vi "Running Wrapper.vi"(8 "error in (no error)":errorcluster, 11 "CIFCorePlugin in":refnum<class "CIFCorePlugin.lvclass">) -> (0 "error out":errorcluster, 2 "Destroy":bool, 3 "CIFCorePlugin out":refnum<class "CIFCorePlugin.lvclass">)   [LabVIEW 2021, in "CIFCorePlugin.lvclass"]
doc: "Wrapper around the Core Running VI. This wrapper will handle selection of timed loop with priorities or execution without a timed loop. \n\nIf the VI is compiled to run on LinuxRT it will check if timed loop is supported (RT compiled PPLs can run on desktop but timed loop is not supported and conditional compile will not check after PPL is compiled). If the timed loop is supported it will check if the priority is a positive value. If positive it will run in timed loop and set priority. A negative value will indicate configuration to not used timed loop."
uses:
  CIFCorePlugin.lvclass
  CIFCorePlugin.lvclass/CIFCorePlugin.ctl
  <vilib>/Platform/TimedLoop/XDataNode/wakeup.ctl
  <vilib>/Platform/TimedLoop/XDataNode/XDNodeRunTimeDep.lvlib
  <vilib>/Platform/TimedLoop/XDataNode/nitl_modes.ctl
  <vilib>/Platform/TimedLoop/XDataNode/timing_clust.ctl
  <vilib>/Platform/TimedLoop/XDataNode/XDataNode.xnode
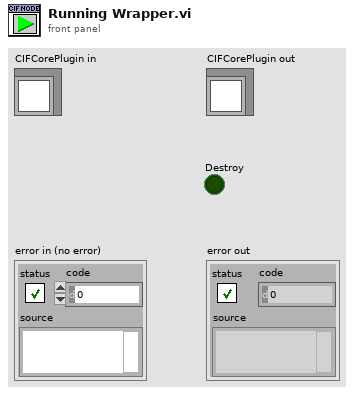
[diagram p1: front panel]
types:
  T1 = typedef "XDNodeRunTimeDep.lvlib/timing_clust.ctl" = cluster{"Expected End [f-1]":u64, "Actual End [f-1]":u64, "Finished Late? [f-1]":bool, "Expected End [i-1]":u64, "Actual End [i-1]":u64, "Finished Late? [i-1]":bool, "Expected Start [i]":u64, "Actual Start [i]":u64, "Expected Start [f]":u64, "Actual Start [f]":u64, "Source Name":string, "Structure Name":string, "Period":i64, "Deadline":i64, "Offset":i64, "Start":i64, "Priority":i32, "Timeout":i32, "Mode":T2, "Wakeup Reason":T3, "Error":errorcluster, "Source Type":string, "Secondary Source Type":string, "Global End Time":u64, "Global Start Time":u64, "Frame Duration":u64, "Iteration Duration":u64, "Assigned CPU":i32, "I/O Scan Engine Mode":u32}
  T2 = typedef "XDNodeRunTimeDep.lvlib/nitl_modes.ctl" = enum32{"No Change", "Process missed periods, maintain original phase", "Discard missed periods, maintain original phase", "Process missed periods, ignore original phase", "Discard missed periods, ignore original phase"}
  T3 = typedef "XDNodeRunTimeDep.lvlib/wakeup.ctl" = enum32{"Normal", "Aborted", "Asynchronous wakeup", "Timing source error", "Timed loop error", "Timeout"}
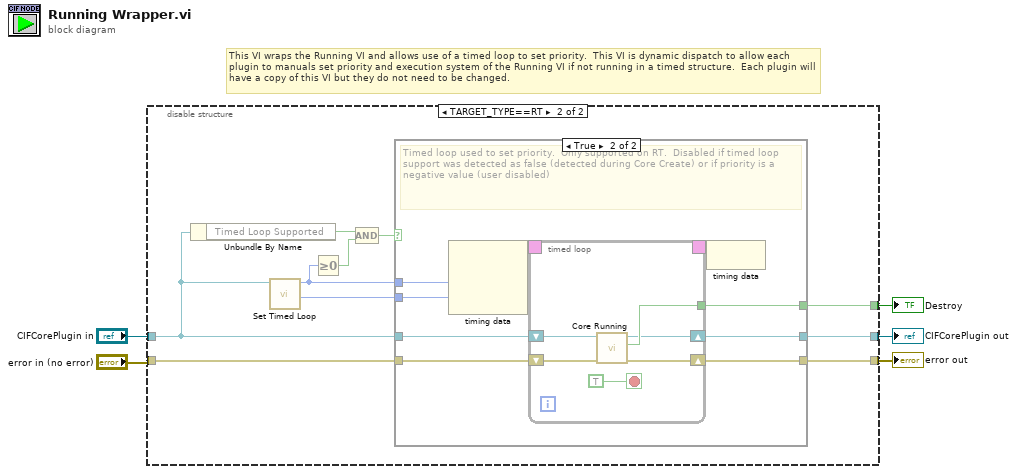
[diagram p0: block diagram]
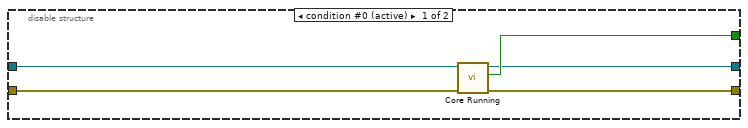
[diagram p2: hidden frame]
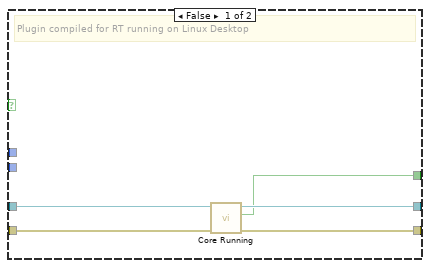
[diagram p3: hidden frame]
diagram:
  # "This VI wraps the Running VI and allows use of a timed loop to set priority.  This VI is dynamic dispatch to allow each plugin to manuals set priority and execution system of the Running VI if not running in a timed structure.  Each plugin will have a copy of this VI but they do not need to be changed."
  n1 = disable-structure shown="TARGET_TYPE==RT" {
    disable-tunnel: "CIFCorePlugin in" -> [w10 w16]
    disable-tunnel: "error in (no error)" -> [w9 w20]
    disable-tunnel: [w8 w19] -> w1
    disable-tunnel: [w7 w18] -> w3
    disable-tunnel: [w6 w17] -> w2
    frame condition #0 (active) {
      n2 = call "Core Running.vi"("error in (no error)"=w9, "CIFCorePlugin in"=w10) -> ("error out"=w6:errorcluster, "Destroy"=w8:bool, "CIFCorePlugin out"=w7:refnum<class "CIFCorePlugin.lvclass">)  [unwired: 7 in]
    }
    frame condition #1 {
      n3 = Unbundle By Name(w16) -> ("Timed Loop Supported"=w13:bool)
      n4 = call "Set Timed Loop.vi"("CIFCorePlugin in"=w16) -> ("Processor"=w15:i32, "Priority"=w14:i32)  [unwired: 9 in]
      n5 = Greater Or Equal To 0?(x=w14) -> (x >= 0?=w12:bool)
      n6 = Compound Arithmetic op=AND(w13, w12) -> (w11:bool)
      n7 = case shown="True" w11 {
        tunnel: w20 -> [w24 w32]
        tunnel: [w21 w31] -> w19
        tunnel: [w23 w30] -> w18
        tunnel: [w22 w29] -> w17
        tunnel: w16 -> [w25 w28]
        tunnel: w14 -> [_ w27]
        tunnel: w15 -> [_ w26]
        frame False {
          # "Plugin compiled for RT running on Linux Desktop"
          n8 = call "Core Running.vi"("error in (no error)"=w24, "CIFCorePlugin in"=w25) -> ("error out"=w22:errorcluster, "Destroy"=w21:bool, "CIFCorePlugin out"=w23:refnum<class "CIFCorePlugin.lvclass">)  [unwired: 7 in]
        }
        frame True {
          # "Timed loop used to set priority.  Only supported on RT.  Disabled if timed loop support was detected as false (detected during Core Create) or if priority is a negative value (user disabled)"
          n9 = node-c288(w27, w26) -> (w34:T1)  [unwired: 1 in]
          n10 = timed-loop {
            timing: w34 -> [_]
            timing-out: [_] -> w33
            shift-right: [w38] -> w30
            shift-left: w28 -> [w36]
            shift-right: [w37] -> w29
            shift-left: w32 -> [w35]
            tunnel: [w39] -> w31
            stop <- TRUE stop-if-true
            n11 = call "Core Running.vi"("error in (no error)"=w35, "CIFCorePlugin in"=w36) -> ("error out"=w37:errorcluster, "Destroy"=w39:bool, "CIFCorePlugin out"=w38:refnum<class "CIFCorePlugin.lvclass">)  [unwired: 7 in]
          }
          n12 = node-c288(w33) -> ()
        }
      }
    }
  }
  "error out" <- w2
  "CIFCorePlugin out" <- w3
  "Destroy" <- w1
